vi "Create New RESTful Web Service.vi"(7 "TargetItem Refnum":refnum<vi>, 8 "error in (no error)":errorcluster, 9 "Build Path":path, 10 "Build specification name":string, 11 "Project Refnum":refnum<vi>) -> (0 "error out":errorcluster, 3 "RESTful out":refnum<class "NI_AB_API_RESTful.lvclass">)   [LabVIEW 2020, in "NI_AB_API_RESTful.lvclass"]
uses:
  <vilib>/AppBuilder/AB_API/RESTful/NI_AB_API_RESTful.lvclass
  <vilib>/AppBuilder/AB_API/RESTful/NI_AB_API_RESTful.lvclass/NI_AB_API_RESTful.ctl
  <vilib>/AppBuilder/AB_API/common/AB_API Build Object Type.ctl
  <vilib>/AppBuilder/AB_API/Build/NI_AB_API_Build.lvclass
  <vilib>/AppBuilder/AB_Classes/RESTful/AB_RESTfulWebService.lvclass
  e:/builds/penguin/labview/branches/2020/dev/dist/vi.lib/AppBuilder/AB_Classes/WebService/AB_WebService.lvclass
  e:/builds/penguin/labview/branches/2020/dev/dist/vi.lib/AppBuilder/AB_Classes/TargetFile/AB_Targetfile.lvclass
  e:/builds/penguin/labview/branches/2020/dev/dist/vi.lib/AppBuilder/AB_Classes/Build/AB_Build.lvclass
  e:/builds/penguin/labview/branches/2020/dev/dist/vi.lib/AppBuilder/AB_Classes/RESTful/AB_RESTfulWebService.lvclass
  e:/builds/penguin/labview/branches/2020/dev/dist/vi.lib/AppBuilder/AB_API/Targetfile/NI_AB_API_Targetfile.lvclass
  e:/builds/penguin/labview/branches/2020/dev/dist/vi.lib/AppBuilder/AB_API/Build/NI_AB_API_Build.lvclass
  e:/builds/penguin/labview/branches/2020/dev/dist/vi.lib/AppBuilder/AB_API/RESTful/NI_AB_API_RESTful.lvclass
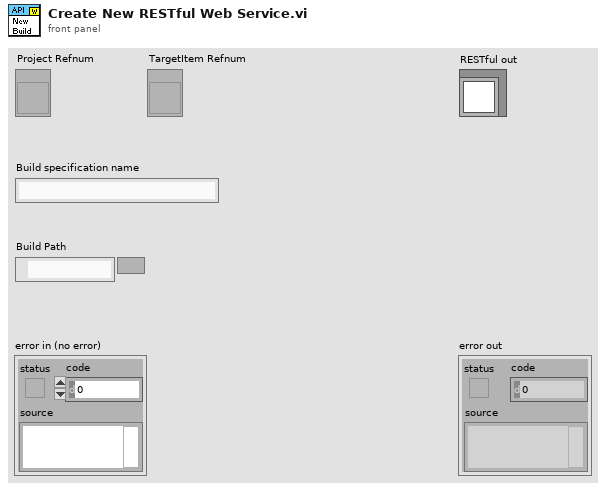
[diagram p1: front panel]
types:
  T1 = typedef "AB_API Build Object Type.ctl" = enum16{"Source Distribution", "DLL", "EXE", "Installer", "Zip File", "RESTful WS", "RTEXE", "Packed Library", "C Generation ", ".NET Interop Assembly"}
  T2 = typedef "ItemRef.ctl" = u64
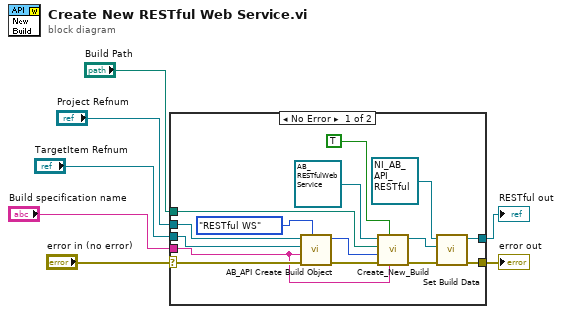
[diagram p0: block diagram]
diagram:
  n1 = case shown="No Error" "error in (no error)" {
    selector: "error in (no error)" -> [w21 w23]
    tunnel: [w9 w23] -> w6
    tunnel: [w10 _] -> w5
    tunnel: "Build specification name" -> [w8 _]
    tunnel: "TargetItem Refnum" -> [w22 _]
    tunnel: "Project Refnum" -> [w19 _]
    tunnel: "Build Path" -> [w11 _]
    frame No Error {
      n2 = call <vilib>:"AB_API Create Build Object.vi"("Build object type"=AB_API_Build_Object_Type."RESTful WS", "error in (no error)"=w21, "Build spec name"=w8, "TargetItem Refnum"=w22, "Project Refnum"=w19) -> ("error out"=w16:errorcluster, "Build object"=w17:T2)  [unwired: 5 in]
      n3 = call-dynamic "Create_New_Build.vi"("buildSpecName"=w8, "Programmatic? (false)"=TRUE, "error in (no error)"=w16, "buildObject"=w17, "Destination Path"=w11, "AB_WebService in"=refnum<class "AB_RESTfulWebService.lvclass"> refnum ("AB_RESTfulWebService.lvclass")) -> ("error out"=w15:errorcluster, "AB_WebService out"=w14:refnum<class "AB_RESTfulWebService.lvclass">)  [unwired: 4 in]
      n4 = call <vilib>:"Set Build Data.vi"("error in (no error)"=w15, "AB_Build.lvclass"=w14, "NI_AB_API_Build in"=refnum<class "NI_AB_API_RESTful.lvclass"> refnum ("AB_API_SDIST.lvclass")) -> ("error out"=w9:errorcluster, "NI_AB_API_Build out"=w10:refnum<class "NI_AB_API_RESTful.lvclass">)  [unwired: 7 in]
    }
    frame Error {
    }
  }
  "error out" <- w6
  "RESTful out" <- w5
